vi "MC5e Parse Squad Cluster to String Array.vi"(11 "Squad Info":T1 {"CR" items=["30", "29", "28", "27", "26", "25", "24", "23", "22", "21", "20", "19", "18", "17", "16", "15", "14", "13", "12", "11", "10", "9", "8", "7", "6", "5", "4", "3", "2", "1", "1/2", "1/4", "1/8"]}) -> (2 "Labeled Array":string[](array[string]), 3 "Array":string[](array[string]))   [LabVIEW 2020]
uses:
  MC5e Squad_Info.ctl
  MC5e Size_Categories.ctl
panel:
  # "Squads are restricted to one type of soldier (i.e  Archers) and all of the same level.\nIf you want mixed CR or mixed types, use multiple squads."
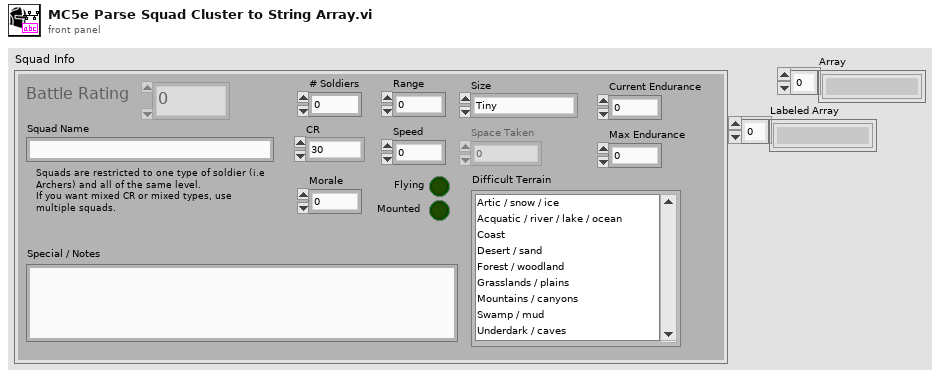
[diagram p1: front panel]
types:
  T1 = typedef "MC5e Squad_Info.ctl" = cluster{"Squad Name":string, "# Soldiers":u16, "Battle Rating":u16, "Flying":bool, "Mounted":bool, "Speed":u16, "Range":u16, "Morale":i32, "Max Endurance":u16, "Current Endurance":i32, "Size":T2, "Space Taken":u16, "Difficult Terrain":i32[], "CR":u16, "Special / Notes":string}
  T2 = typedef "MC5e Size_Categories.ctl" = enum16{"Tiny", "Small", "Medium", "Large", "Huge", "Gargantuan"}
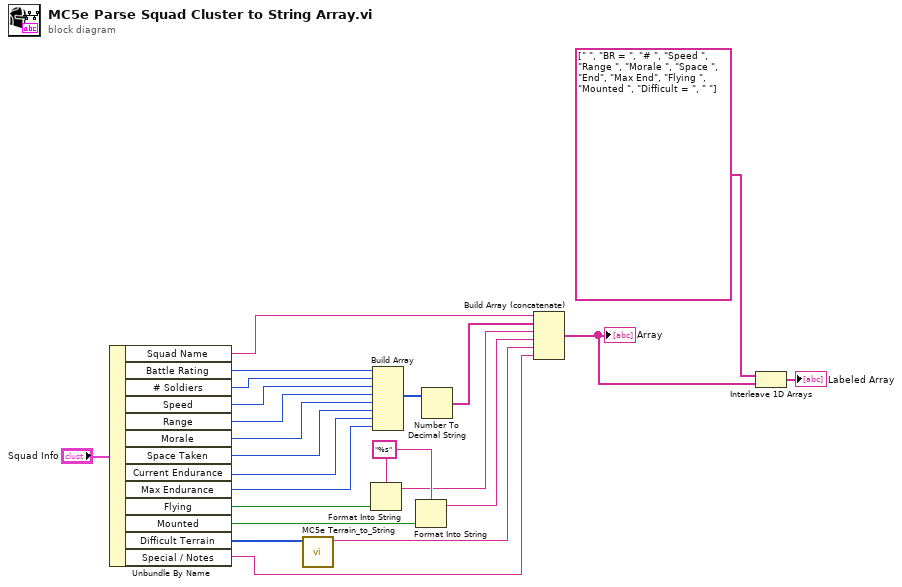
[diagram p0: block diagram]
diagram:
  w18 = "%s" ("format string")
  n1 = Unbundle By Name("Squad Info") -> ("Squad Name"=w23:string, "Battle Rating"=w22:u16, "# Soldiers"=w20:u16, "Speed"=w5:u16, "Range"=w6:u16, "Morale"=w7:i32, "Space Taken"=w21:u16, "Current Endurance"=w8:i32, "Max Endurance"=w9:u16, "Flying"=w11:bool, "Mounted"=w12:bool, "Difficult Terrain"=w13:i32[], "Special / Notes"=w17:string)
  n2 = call "MC5e Terrain_to_String.vi"("Difficult Terrain"=w13) -> ("Difficult Terrain String"=w16:string)  [unwired: 10 in]
  n3 = Format Into String(format string=w18, w11) -> (resulting string=w15:string)  [unwired: 2 in, 1 out]
  n4 = Build Array(w22, w20, w5, w6, w7, w21, w8, w9) -> (w10:i32[])
  n5 = Format Into String(format string=w18, w12) -> (resulting string=w19:string)  [unwired: 2 in, 1 out]
  n6 = Number To Decimal String(number=w10) -> (decimal integer string=w14:string[])  [unwired: 1 in]
  n7 = Build Array (concatenate)(w23, w14, w15, w19, w16, w17) -> (w3:string[])
  "Array" <- w3
  n8 = Interleave 1D Arrays(string[] [" ", "BR = ", "# ", "Speed ", "Range ", "Morale ", "Space ", "End", "Max End", "Flying ", "Mounted ", "Difficult = ", " "] ("appended array"), w3) -> (→"Labeled Array":string[])
